vi "Tri-Tri minimum separation.vi"(2 "Triangle 2":T1, 3 "Triangle 1":T1) -> (0 "Minimum separation distance":sgl, 1 "Minimum separation vector\nfrom triangle 2 to triange 1":sgl[](array[numeric]))   [LabVIEW 2014]
uses:
  Typedefs/Triangle.ctl
panel:
  # "PN 13/01/2015"
  # "Vertices"
  # "Edges"
  # "Unit normal"
  # "pre-store"
  # "Vertices"
  # "Edges"
  # "Unit normal"
  # "pre-store"
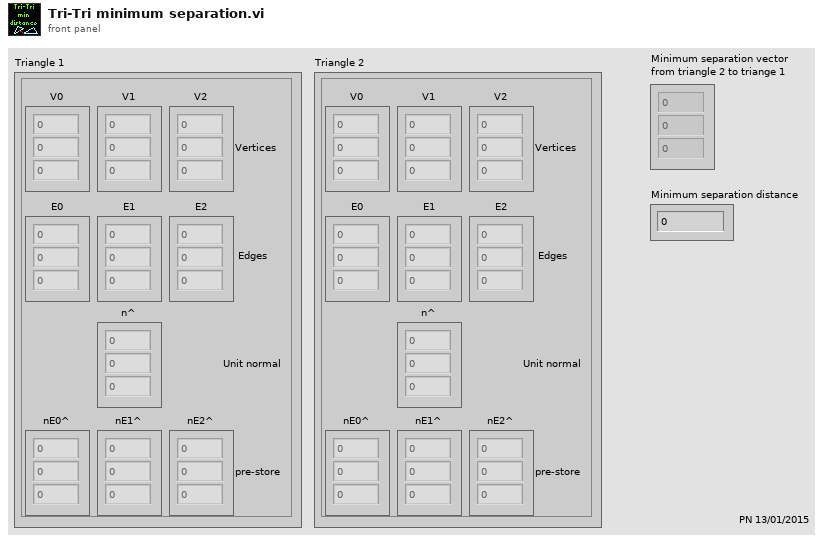
[diagram p1: front panel]
types:
  T1 = typedef "Triangle.ctl" = cluster{"V0":sgl[], "V1":sgl[], "V2":sgl[], "E0":sgl[], "E1":sgl[], "E2":sgl[], "n^":sgl[], "nE0^":sgl[], "nE1^":sgl[], "nE2^":sgl[]}
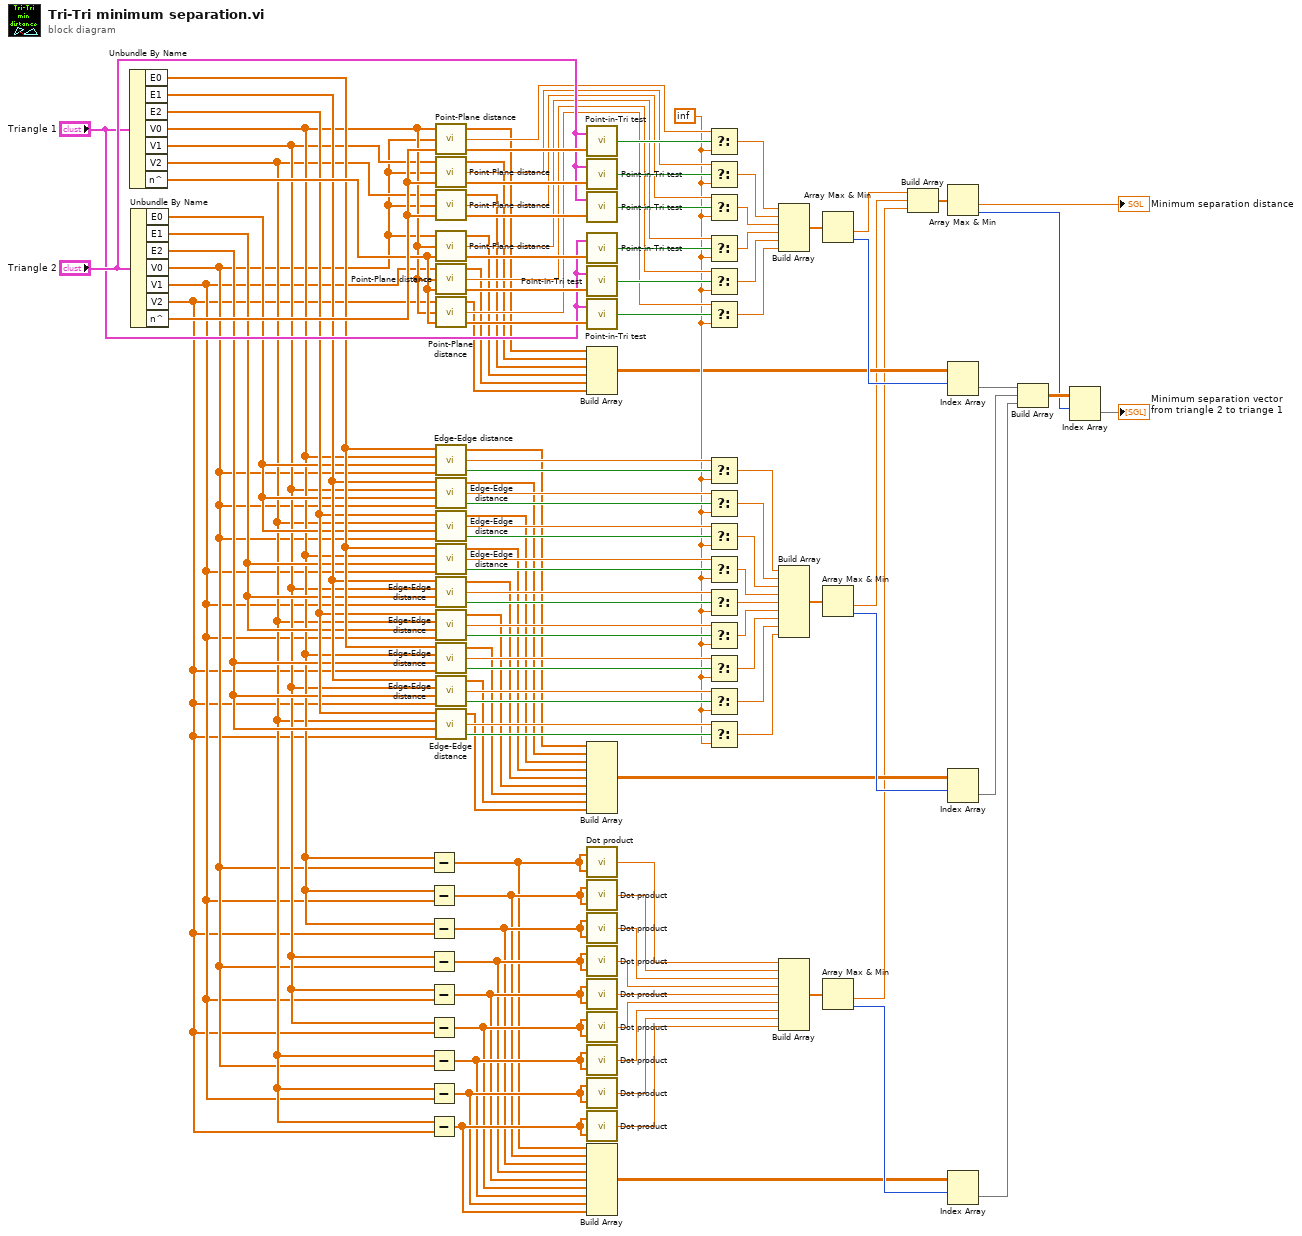
[diagram p0: block diagram]
diagram:
  w75 = sgl inf
  n1 = Unbundle By Name("Triangle 1") -> ("E0"=w111:sgl[], "E1"=w110:sgl[], "E2"=w109:sgl[], "V0"=w74:sgl[], "V1"=w73:sgl[], "V2"=w72:sgl[], "n^"=w112:sgl[])
  n2 = Unbundle By Name("Triangle 2") -> ("E0"=w108:sgl[], "E1"=w107:sgl[], "E2"=w106:sgl[], "V0"=w71:sgl[], "V1"=w70:sgl[], "V2"=w69:sgl[], "n^"=w120:sgl[])
  n3 = Subtract(x=w74, y=w71) -> (x-y=w60:sgl[])
  n4 = Subtract(x=w74, y=w70) -> (x-y=w61:sgl[])
  n5 = Subtract(x=w74, y=w69) -> (x-y=w62:sgl[])
  n6 = Subtract(x=w73, y=w71) -> (x-y=w63:sgl[])
  n7 = Subtract(x=w73, y=w70) -> (x-y=w64:sgl[])
  n8 = Subtract(x=w73, y=w69) -> (x-y=w65:sgl[])
  n9 = Subtract(x=w72, y=w71) -> (x-y=w66:sgl[])
  n10 = Subtract(x=w72, y=w70) -> (x-y=w67:sgl[])
  n11 = Subtract(x=w72, y=w69) -> (x-y=w68:sgl[])
  n12 = call "Point-Plane distance.vi"("Plane normal (unit)"=w120, "Point on plane"=w71, "Point"=w74) -> ("Projected point on plane (along normal)"=w121:sgl[], "| Distance |"=w99:sgl, "Distance vector"=w45:sgl[])
  n13 = call "Point-Plane distance.vi"("Plane normal (unit)"=w120, "Point on plane"=w71, "Point"=w73) -> ("Projected point on plane (along normal)"=w119:sgl[], "| Distance |"=w98:sgl, "Distance vector"=w46:sgl[])
  n14 = call "Point-Plane distance.vi"("Plane normal (unit)"=w120, "Point on plane"=w71, "Point"=w72) -> ("Projected point on plane (along normal)"=w118:sgl[], "| Distance |"=w97:sgl, "Distance vector"=w47:sgl[])
  n15 = call "Point-Plane distance.vi"("Plane normal (unit)"=w112, "Point on plane"=w74, "Point"=w71) -> ("Projected point on plane (along normal)"=w114:sgl[], "| Distance |"=w96:sgl, "Distance vector"=w48:sgl[])
  n16 = call "Point-Plane distance.vi"("Plane normal (unit)"=w112, "Point on plane"=w74, "Point"=w70) -> ("Projected point on plane (along normal)"=w115:sgl[], "| Distance |"=w95:sgl, "Distance vector"=w49:sgl[])
  n17 = call "Point-Plane distance.vi"("Plane normal (unit)"=w112, "Point on plane"=w74, "Point"=w69) -> ("Projected point on plane (along normal)"=w116:sgl[], "| Distance |"=w94:sgl, "Distance vector"=w50:sgl[])
  n18 = call "Edge-Edge distance.vi"("Edge 2 start point"=w71, "Edge 2 (not unit)"=w108, "Edge 1 start point"=w74, "Edge 1 (not unit)"=w111) -> ("Include"=w93:bool, "Distance^2"=w87:sgl, "Distance vector"=w51:sgl[])
  n19 = call "Edge-Edge distance.vi"("Edge 2 start point"=w71, "Edge 2 (not unit)"=w108, "Edge 1 start point"=w73, "Edge 1 (not unit)"=w110) -> ("Include"=w92:bool, "Distance^2"=w86:sgl, "Distance vector"=w52:sgl[])
  n20 = call "Edge-Edge distance.vi"("Edge 2 start point"=w71, "Edge 2 (not unit)"=w108, "Edge 1 start point"=w72, "Edge 1 (not unit)"=w109) -> ("Include"=w91:bool, "Distance^2"=w85:sgl, "Distance vector"=w53:sgl[])
  n21 = call "Edge-Edge distance.vi"("Edge 2 start point"=w70, "Edge 2 (not unit)"=w107, "Edge 1 start point"=w74, "Edge 1 (not unit)"=w111) -> ("Include"=w90:bool, "Distance^2"=w84:sgl, "Distance vector"=w54:sgl[])
  n22 = call "Edge-Edge distance.vi"("Edge 2 start point"=w70, "Edge 2 (not unit)"=w107, "Edge 1 start point"=w73, "Edge 1 (not unit)"=w110) -> ("Include"=w89:bool, "Distance^2"=w83:sgl, "Distance vector"=w55:sgl[])
  n23 = call "Edge-Edge distance.vi"("Edge 2 start point"=w70, "Edge 2 (not unit)"=w107, "Edge 1 start point"=w72, "Edge 1 (not unit)"=w109) -> ("Include"=w88:bool, "Distance^2"=w82:sgl, "Distance vector"=w56:sgl[])
  n24 = call "Edge-Edge distance.vi"("Edge 2 start point"=w69, "Edge 2 (not unit)"=w106, "Edge 1 start point"=w74, "Edge 1 (not unit)"=w111) -> ("Include"=w81:bool, "Distance^2"=w78:sgl, "Distance vector"=w57:sgl[])
  n25 = call "Edge-Edge distance.vi"("Edge 2 start point"=w69, "Edge 2 (not unit)"=w106, "Edge 1 start point"=w73, "Edge 1 (not unit)"=w110) -> ("Include"=w80:bool, "Distance^2"=w77:sgl, "Distance vector"=w58:sgl[])
  n26 = call "Edge-Edge distance.vi"("Edge 2 start point"=w69, "Edge 2 (not unit)"=w106, "Edge 1 start point"=w72, "Edge 1 (not unit)"=w109) -> ("Include"=w79:bool, "Distance^2"=w76:sgl, "Distance vector"=w59:sgl[])
  n27 = call "Point-in-Tri test.vi"("Point"=w121, "Triangle"="Triangle 2") -> ("Point is inside triangle"=w105:bool)
  n28 = call "Point-in-Tri test.vi"("Point"=w119, "Triangle"="Triangle 2") -> ("Point is inside triangle"=w104:bool)
  n29 = call "Point-in-Tri test.vi"("Point"=w118, "Triangle"="Triangle 2") -> ("Point is inside triangle"=w103:bool)
  n30 = call "Point-in-Tri test.vi"("Point"=w114, "Triangle"="Triangle 1") -> ("Point is inside triangle"=w102:bool)
  n31 = call "Point-in-Tri test.vi"("Point"=w115, "Triangle"="Triangle 1") -> ("Point is inside triangle"=w101:bool)
  n32 = call "Point-in-Tri test.vi"("Point"=w116, "Triangle"="Triangle 1") -> ("Point is inside triangle"=w100:bool)
  n33 = Build Array(w45, w46, w47, w48, w49, w50) -> (w12:sgl[][])
  n34 = Build Array(w51, w52, w53, w54, w55, w56, w57, w58, w59) -> (w18:sgl[][])
  n35 = call "Dot product.vi"("B"=w60, "A"=w60) -> ("A . B"=w29:sgl)
  n36 = call "Dot product.vi"("B"=w61, "A"=w61) -> ("A . B"=w28:sgl)
  n37 = call "Dot product.vi"("B"=w62, "A"=w62) -> ("A . B"=w27:sgl)
  n38 = call "Dot product.vi"("B"=w63, "A"=w63) -> ("A . B"=w26:sgl)
  n39 = call "Dot product.vi"("B"=w64, "A"=w64) -> ("A . B"=w25:sgl)
  n40 = call "Dot product.vi"("B"=w65, "A"=w65) -> ("A . B"=w24:sgl)
  n41 = call "Dot product.vi"("B"=w66, "A"=w66) -> ("A . B"=w21:sgl)
  n42 = call "Dot product.vi"("B"=w67, "A"=w67) -> ("A . B"=w22:sgl)
  n43 = call "Dot product.vi"("B"=w68, "A"=w68) -> ("A . B"=w23:sgl)
  n44 = Build Array(w60, w61, w62, w63, w64, w65, w66, w67, w68) -> (w15:sgl[][])
  n45 = Select(t=w99, s=w105, f=w75) -> (s? t:f=w44:sgl)
  n46 = Select(t=w98, s=w104, f=w75) -> (s? t:f=w43:sgl)
  n47 = Select(t=w97, s=w103, f=w75) -> (s? t:f=w42:sgl)
  n48 = Select(t=w96, s=w102, f=w75) -> (s? t:f=w41:sgl)
  n49 = Select(t=w95, s=w101, f=w75) -> (s? t:f=w40:sgl)
  n50 = Select(t=w94, s=w100, f=w75) -> (s? t:f=w39:sgl)
  n51 = Select(t=w87, s=w93, f=w75) -> (s? t:f=w38:sgl)
  n52 = Select(t=w86, s=w92, f=w75) -> (s? t:f=w37:sgl)
  n53 = Select(t=w85, s=w91, f=w75) -> (s? t:f=w36:sgl)
  n54 = Select(t=w84, s=w90, f=w75) -> (s? t:f=w35:sgl)
  n55 = Select(t=w83, s=w89, f=w75) -> (s? t:f=w34:sgl)
  n56 = Select(t=w82, s=w88, f=w75) -> (s? t:f=w33:sgl)
  n57 = Select(t=w78, s=w81, f=w75) -> (s? t:f=w32:sgl)
  n58 = Select(t=w77, s=w80, f=w75) -> (s? t:f=w31:sgl)
  n59 = Select(t=w76, s=w79, f=w75) -> (s? t:f=w30:sgl)
  n60 = Build Array(w44, w43, w42, w41, w40, w39) -> (w13:sgl[])
  n61 = Build Array(w38, w37, w36, w35, w34, w33, w32, w31, w30) -> (w20:sgl[])
  n62 = Build Array(w29, w28, w27, w26, w25, w24, w21, w22, w23) -> (w17:sgl[])
  n63 = Array Max & Min(array=w13) -> (min value=w11:sgl, min index (indices)=w14:i32)  [unwired: 2 out]
  n64 = Array Max & Min(array=w20) -> (min value=w10:sgl, min index (indices)=w19:i32)  [unwired: 2 out]
  n65 = Array Max & Min(array=w17) -> (min value=w9:sgl, min index (indices)=w16:i32)  [unwired: 2 out]
  n66 = Build Array(w11, w10, w9) -> (w5:sgl[])
  n67 = Array Max & Min(array=w5) -> (min value=→"Minimum separation distance":sgl, min index (indices)=w3:i32)  [unwired: 2 out]
  n68 = Index Array(array=w12, index (row)=w14) -> (element=w6:sgl[])  [unwired: 1 in]
  n69 = Index Array(array=w18, index (row)=w19) -> (element=w8:sgl[])  [unwired: 1 in]
  n70 = Index Array(array=w15, index (row)=w16) -> (element=w7:sgl[])  [unwired: 1 in]
  n71 = Build Array(w6, w8, w7) -> (w4:sgl[][])
  n72 = Index Array(array=w4, index (row)=w3) -> (element=→"Minimum separation vector\nfrom triangle 2 to triange 1":sgl[])  [unwired: 1 in]
